vi "projVTOL.vi"() -> ()   [LabVIEW 2022 SP3]
uses:
  <vilib>/Utility/error.llb/Trim Whitespace One-Sided.vi
  <vilib>/Instr/_visa.llb/VISA Configure Serial Port (Instr).vi
panel:
  in  "stop":bool
  in  "Start":bool
  in  "Tab Control":T1(tab)
  in  "Nb octets à lire":u16
  in  "VISA resource name":refnum<visa-resource-name>
  in  "baud rate (9600)":u32=9600
  in  "data bits (8)":u16=8 min=5 max=8 step=1
  in  "parity (0:none)":enum16{"None", "Odd", "Even", "Mark", "Space"}(ring)
  in  "termination char\n(0xA = '\\n' = LF)":u8=10 format="%.0x"
  in  "Enable Termination\nChar (T)":bool=TRUE
  in  "Erreur écriture":errorcluster
  in  "Erreur fermeture":errorcluster
  out "Données reçues (chaine)":string
  out "Tableau des données reçues":dbl[](array[numeric])
  in  "Ki":dbl(slide) scale=0.0..20.0
  in  "Kd":dbl(slide) scale=0.0..20.0
  in  "Kp":dbl(slide) scale=0.0..200.0
  in  "Lire les données":bool
  in  "Transmettre les données":bool
  in  "Consigne":dbl(knob) scale=-20.0..20.0
  in  "Erreur ouvrir/remplacer/créer fichier":errorcluster
  out "Equilibre atteint":bool
  out "Position angulaire":cluster{dbl, "Consigne":dbl}(graph)
  out "Vitesse angulaire":dynamicdata(graph)
  out "Accéleration":dynamicdata(graph)
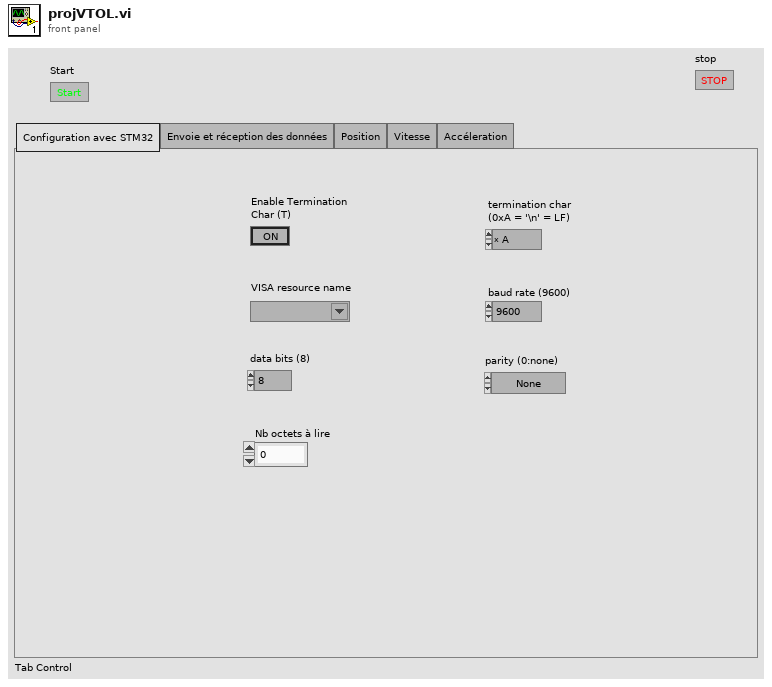
[diagram p1: front panel]
types:
  T1 = enum32{"Configuration avec STM32", "Envoie et réception des données", "Position", "Vitesse", "Accéleration"}
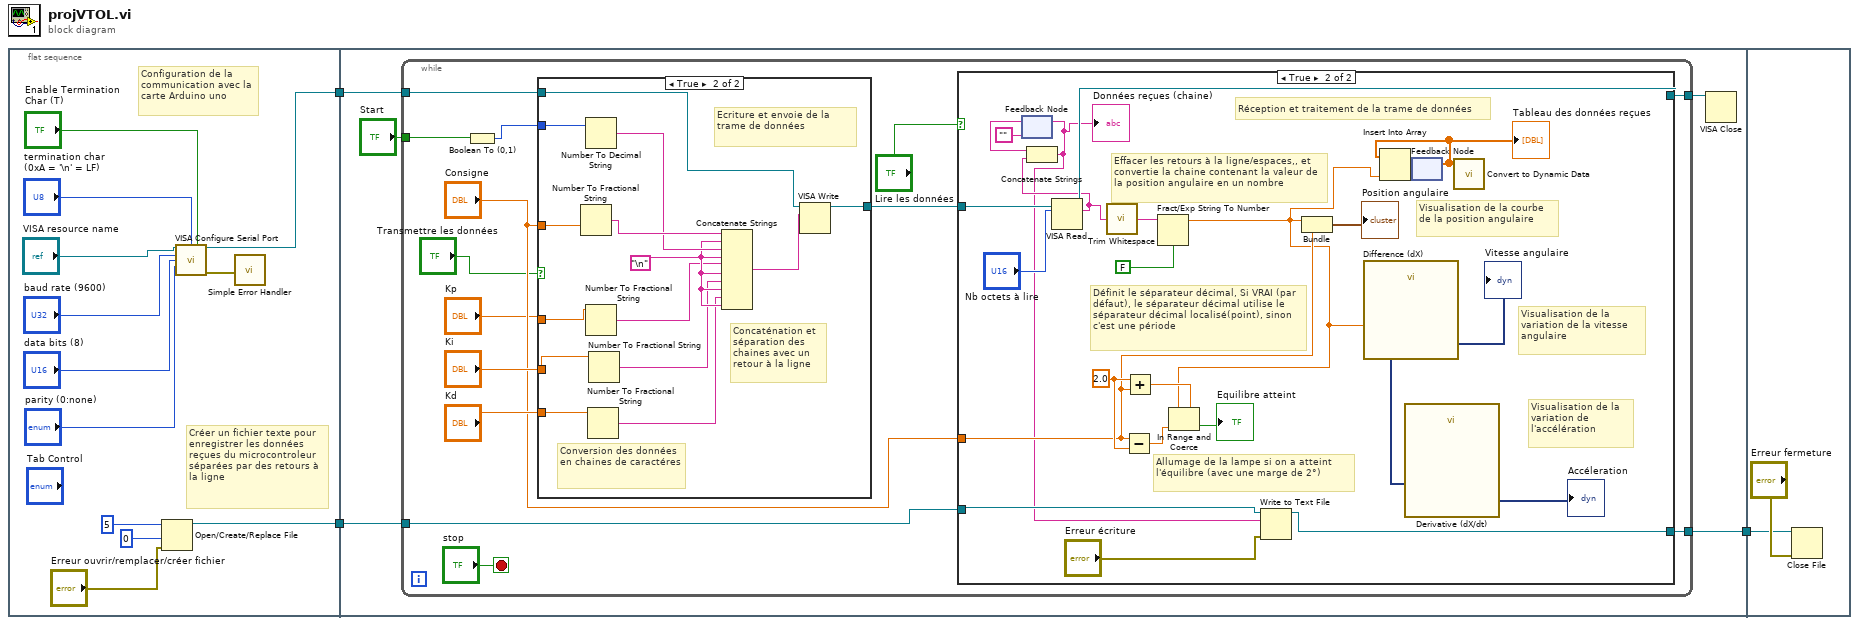
[diagram p0: block diagram]
diagram:
  n1 = flat-sequence {
    tunnel: [w5] -> w3
    tunnel: [w4] -> w2
    tunnel: w3 -> [w19]
    tunnel: w2 -> [w18]
    tunnel: [w17] -> w1
    tunnel: w1 -> [w75]
    frame #0 {
      # "Créer un fichier texte pour enregistrer les données reçues du microcontroleur séparées par des retours à la ligne"
      # "Configuration de la communication avec la carte Arduino uno"
      n2 = Open/Create/Replace File(error in="Erreur ouvrir/remplacer/créer fichier", operation (0:open)=5, access (0:read/write)=0) -> (refnum out=w4:refnum<file>)  [unwired: 3 in, 2 out]
      n3 = call-poly "VISA Configure Serial Port"("VISA resource name"="VISA resource name", "termination char\n(0xA = '\\n' = LF)"="termination char\n(0xA = '\\n' = LF)", "Enable Termination\nChar (T)"="Enable Termination\nChar (T)", "baud rate (9600)"="baud rate (9600)", "data bits (8)"="data bits (8)", "parity (0:none)"="parity (0:none)") -> ("VISA resource name out"=w5:refnum<visa-resource-name>, "error out"=w9:errorcluster)  [unwired: 8 in]
      n4 = call <vilib>:"Simple Error Handler.vi"("error in (no error)"=w9) -> ()  [unwired: 4 in, 5 out]
    }
    frame #1 {
      n5 = while {
        tunnel: "Start" -> [w29]
        tunnel: w19 -> [w32]
        tunnel: w18 -> [w27]
        tunnel: [w26] -> w17
        tunnel: [w21] -> w16
        stop <- "stop" stop-if-true
        n6 = Boolean To (0,1)(Boolean=w29) -> (0, 1=w33:i16)
        n7 = case shown="True" "Transmettre les données" {
          tunnel: w33 -> [_ w74]
          tunnel: w32 -> [w60 w72]
          tunnel: "Consigne" -> [_ w71]
          tunnel: "Kp" -> [_ w70]
          tunnel: "Ki" -> [_ w61]
          tunnel: "Kd" -> [_ w69]
          tunnel: [w60 w62] -> w28
          frame False {
          }
          frame True {
            w66 = "\n"
            # "Ecriture et envoie de la trame de données"
            # "Concaténation et séparation des chaines avec un retour à la ligne"
            # "Conversion des données en chaines de caractéres"
            n8 = Number To Fractional String(number=w71) -> (F-format string=w68:string)  [unwired: 3 in]
            n9 = Number To Decimal String(number=w74) -> (decimal integer string=w67:string)  [unwired: 1 in]
            n10 = Number To Fractional String(number=w70) -> (F-format string=w65:string)  [unwired: 3 in]
            n11 = Number To Fractional String(number=w69) -> (F-format string=w63:string)  [unwired: 3 in]
            n12 = Number To Fractional String(number=w61) -> (F-format string=w64:string)  [unwired: 3 in]
            n13 = Concatenate Strings(w68, w66, w67, w66, w65, w66, w64, w66, w63, w66) -> (w73:string)
            n14 = VISA Write(VISA resource name=w72, write buffer=w73) -> (VISA resource name out=w62:refnum<visa-resource-name>)  [unwired: 1 in, 2 out]
          }
        }
        n15 = case shown="True" "Lire les données" {
          tunnel: w28 -> [w35 w59]
          tunnel: w27 -> [w36 w51]
          tunnel: [w36 w50] -> w26
          tunnel: "Consigne" -> [_ w48]
          tunnel: [w35 w46] -> w21
          frame False {
          }
          frame True {
            w54 = 2.0
            # "Visualisation de la variation de l'accélération"
            # "Visualisation de la variation de la vitesse angulaire"
            # "Visualisation de la courbe de la position angulaire"
            # "Allumage de la lampe si on a atteint l'équilibre (avec une marge de 2°)"
            # "Définit le séparateur décimal, Si VRAI (par défaut), le séparateur décimal utilise le séparateur décimal localisé(point), sinon c'est une période"
            # "Effacer les retours à la ligne/espaces,, et convertie la chaine contenant la valeur de la position angulaire en un nombre"
            # "Réception et traitement de la trame de données"
            n16 = feedback #1("") -> (w45:string)
            n17 = VISA Read(VISA resource name=w59, byte count="Nb octets à lire") -> (VISA resource name out=w46:refnum<visa-resource-name>, read buffer=w43:string)  [unwired: 1 in, 2 out]
            n18 = Concatenate Strings(w45, w43) -> (w42:string)
            "Données reçues (chaine)" <- w42
            n19 = feedback-in #1(w42) -> ()
            n20 = call <vilib>:"Trim Whitespace.vi"("string"=w43) -> ("trimmed string"=w41:string)  [unwired: 1 in]
            n21 = Subtract(x=w48, y=w54) -> (x-y=w55:dbl)
            n22 = Add(x=w54, y=w48) -> (x+y=w57:dbl)
            n23 = Fract/Exp String To Number(use system decimal point (T)=FALSE, string=w41) -> (number=w37:dbl)  [unwired: 2 in, 1 out]
            n24 = In Range and Coerce(upper limit=w57, x=w37, lower limit=w55) -> (In Range?=→"Equilibre atteint":bool)  [unwired: 1 out]
            n25 = Write to Text File(file (use dialog)=w51, text=w42, error in="Erreur écriture") -> (refnum out=w50:refnum<file>)  [unwired: 1 in, 2 out]
            n26 = Bundle(w37, "Consigne"=w48) -> (→"Position angulaire":cluster{dbl, "Consigne":dbl})  [unwired: 1 in]
            n27 = call "Difference (dX)"("Signals"=w37) -> ("Result"=w38:dynamicdata)  [unwired: 5 in, 1 out]
            "Vitesse angulaire" <- w38
            n28 = call "Derivative (dX/dt)"("Signals"=w38) -> ("Result"=→"Accéleration":dynamicdata)  [unwired: 5 in, 1 out]
            n29 = feedback #2() -> (w39:dbl[])  [unwired: 1 in]
            "Tableau des données reçues" <- w39
            n30 = Insert Into Array(array=w39, new element=w37) -> (w40:dbl[])  [unwired: 1 in]
            n31 = feedback-in #2(w40) -> ()
            n32 = call "Convert to Dynamic Data"("Array"=w39) -> ()  [unwired: 3 in, 1 out]
          }
        }
      }
      n33 = VISA Close(VISA resource name=w16) -> ()  [unwired: 1 in, 1 out]
    }
    frame #2 {
      n34 = Close File(refnum=w75, error in="Erreur fermeture") -> ()  [unwired: 2 out]
    }
  }
